vi "Index Group.vi"(8 "error in (no error)":errorcluster, 11 "bt_Blackboard_Leaf Type in":refnum<class "bt_Blackboard_Leaf Type.lvclass">) -> (0 "error out":errorcluster, 3 "bt_Blackboard_Leaf Type out":refnum<class "bt_Blackboard_Leaf Type.lvclass">)   [LabVIEW 2021]
uses:
  bt_Blackboard_Leaf Type.lvclass
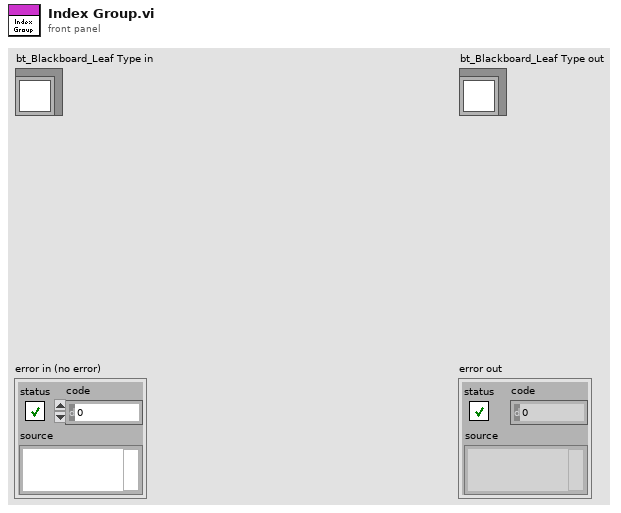
[diagram p1: front panel]
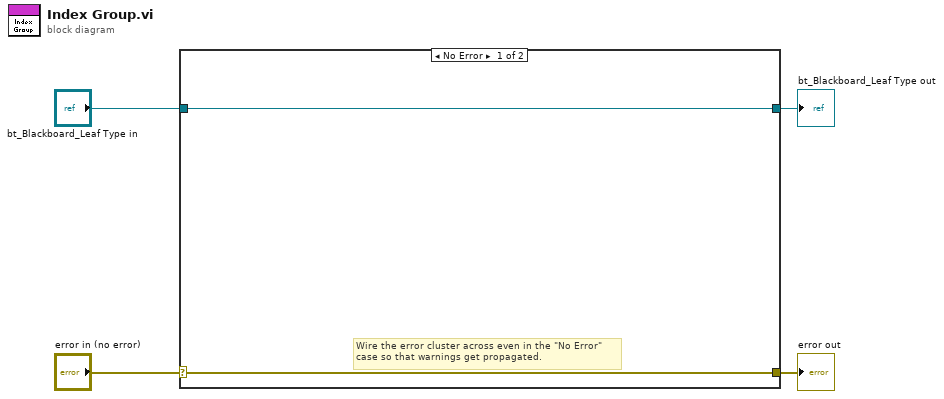
[diagram p0: block diagram]
diagram:
  n1 = case shown="No Error" "error in (no error)" {
    selector: "error in (no error)" -> [w5 w8]
    tunnel: [w5 w8] -> w3
    tunnel: [w6 w7] -> w1
    tunnel: "bt_Blackboard_Leaf Type in" -> [w6 w7]
    frame No Error {
      # "Wire the error cluster across even in the \"No Error\"\ncase so that warnings get propagated."
    }
    frame Error {
    }
  }
  "error out" <- w3
  "bt_Blackboard_Leaf Type out" <- w1
